vi "HGrid_Create.vi"(0 "reference in":refnum<class "HGrid.lvclass">, 5 "error in (no error)":errorcluster) -> (14 "reference out":refnum<class "HGrid.lvclass">, 19 "error out":errorcluster)   [LabVIEW 2019, in "HGrid.lvclass"]
uses:
  HGrid.lvclass
  C:/Users/Taylor.Hillegeist/OneDrive - Ultra/LabVIEW/Pgui2/Pgui_Obj_class/Pgui_Obj.lvclass
  Pgui_Obj_class/Pgui_Obj.lvclass
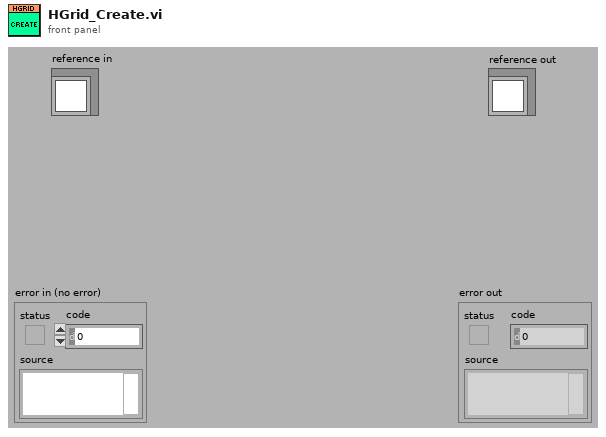
[diagram p1: front panel]
types:
  T1 = typedef "G4SubTemplate_Simple_6x8x6.lvclass/ObjectAttributes.ctl" = cluster{"Attribute1":dbl}
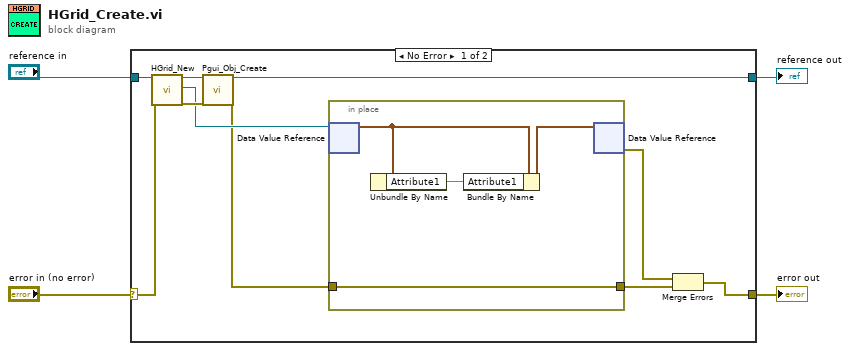
[diagram p0: block diagram]
diagram:
  n1 = case shown="No Error" "error in (no error)" {
    selector: "error in (no error)" -> [w13 w20]
    tunnel: [w11 w20] -> w3
    tunnel: "reference in" -> [w14 w19]
    tunnel: [w8 w19] -> w1
    frame No Error {
      n2 = call "HGrid_New.vi"("reference in"=w14, "error in (no error)"=w13) -> ("reference out"=w10:refnum<class "HGrid.lvclass">, "DVRRefOut"=w7:refnum<data-value>, "error out"=w9:errorcluster)  [unwired: 14 in, 1 out]
      n3 = call "Pgui_Obj_Create.vi"("reference in"=w10, "error in (no error)"=w9) -> ("reference out"=w8:refnum<class "HGrid.lvclass">, "error out"=w6:errorcluster)  [unwired: 16 in]
      n4 = in-place {
        in-place-border: w6 -> [w15]
        in-place-border: [w15] -> w5
        n5 = in-place-dvr #1(w7) -> (w17:T1)  [unwired: 1 out]
        n6 = Unbundle By Name(w17) -> ("Attribute1"=w16:dbl)
        n7 = Bundle By Name(cluster=w17, "Attribute1"=w16) -> (w18:T1)
        n8 = in-place-dvr #1(w18) -> (w12:errorcluster)  [unwired: 1 out]
      }
      n9 = Merge Errors(w12, w5) -> (w11:errorcluster)
    }
    frame Error {
    }
  }
  "error out" <- w3
  "reference out" <- w1
